vi "Write Data.vi"(8 "error in (no error)":errorcluster, 10 "Data":variant, 11 "Expansion in":refnum<class "Expansion.lvclass">) -> (0 "error out":errorcluster, 3 "Expansion out":refnum<class "Expansion.lvclass">)   [LabVIEW 2017, in "Expansion.lvclass"]
uses:
  Expansion.lvclass
  Expansion.lvclass/Expansion.ctl
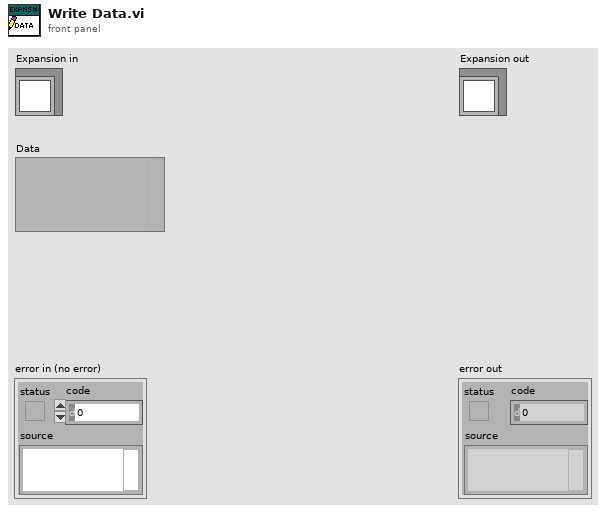
[diagram p1: front panel]
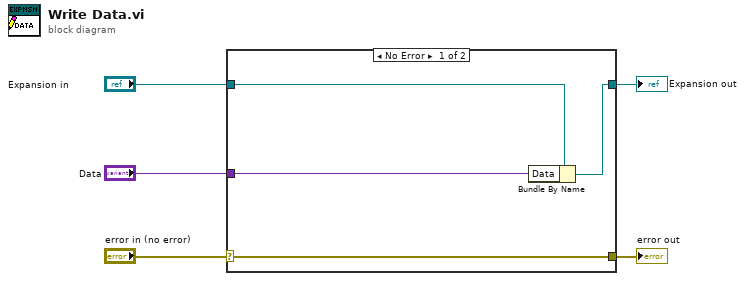
[diagram p0: block diagram]
diagram:
  n1 = case shown="No Error" "error in (no error)" {
    selector: "error in (no error)" -> [w9 w10]
    tunnel: [w9 w10] -> w4
    tunnel: [w7 w11] -> w2
    tunnel: "Expansion in" -> [w8 w11]
    tunnel: "Data" -> [w6 _]
    frame No Error {
      n2 = Bundle By Name(cluster=w8, "Data"=w6) -> (w7:refnum<class "Expansion.lvclass">)
    }
    frame Error {
    }
  }
  "error out" <- w4
  "Expansion out" <- w2
